vi "configure_tx_transfer_group.vi"(7 "Number of Groups":u16, 9 "Channels/Group":u16, 10 "Remote RDMA IP Address":string, 11 "Local RDMA IP Address":string) -> (3 "DSF Configuration":T1)   [LabVIEW 2020]
uses:
  <vilib>/addons/VeriStand Custom Device Scripting APIs/Data Sharing Framework/DSF Core.lvlibp/Typedefs/DSF Settings Info.ctl
  <vilib>/addons/VeriStand Custom Device Scripting APIs/Data Sharing Framework/DSF Core.lvlibp
  <vilib>/addons/VeriStand Custom Device Scripting APIs/Data Sharing Framework/DSF Core.lvlibp/Typedefs/DSF Data Type.ctl
  <vilib>/addons/VeriStand Custom Device Scripting APIs/Data Sharing Framework/DSF Core.lvlibp/Typedefs/Core Channel Configuration.ctl
  <vilib>/addons/VeriStand Custom Device Scripting APIs/Data Sharing Framework/DSF Core.lvlibp/Classes/Configuration/Core/Channel/Channel Configuration.lvclass
  <vilib>/addons/VeriStand Custom Device Scripting APIs/Data Sharing Framework/DSF Core.lvlibp/Typedefs/DSF Engine Channel Configuration.ctl
  <vilib>/addons/VeriStand Custom Device Scripting APIs/Data Sharing Framework/DSF Core.lvlibp/Typedefs/Core Transfer Configuration.ctl
  <vilib>/addons/VeriStand Custom Device Scripting APIs/Data Sharing Framework/DSF Core.lvlibp/Classes/Configuration/Core/Transfer/Transfer Configuration.lvclass
  <vilib>/addons/VeriStand Custom Device Scripting APIs/Data Sharing Framework/DSF Core.lvlibp/Typedefs/DSF Engine Transfer Configuration.ctl
  <vilib>/addons/VeriStand Custom Device Scripting APIs/Data Sharing Framework/DSF Core.lvlibp/Typedefs/DSF Timeout Behavior.ctl
  <vilib>/addons/VeriStand Custom Device Scripting APIs/Data Sharing Framework/DSF Core.lvlibp/Typedefs/DSF Timing Info.ctl
  <vilib>/addons/VeriStand Custom Device Scripting APIs/Data Sharing Framework/DSF Core.lvlibp/Typedefs/DSF Direction.ctl
  <vilib>/addons/VeriStand Custom Device Scripting APIs/Data Sharing Framework/DSF Core.lvlibp/Typedefs/Core Group Configuration.ctl
  <vilib>/addons/VeriStand Custom Device Scripting APIs/Data Sharing Framework/DSF Core.lvlibp/Classes/Configuration/Core/Group/Group Configuration.lvclass
  <vilib>/addons/VeriStand Custom Device Scripting APIs/Data Sharing Framework/DSF Core.lvlibp/Typedefs/DSF Engine Transfer Group Configuration.ctl
  <vilib>/addons/VeriStand Custom Device Scripting APIs/Data Sharing Framework/DSF Core.lvlibp/Typedefs/Core Thread Configuration.ctl
  <vilib>/addons/VeriStand Custom Device Scripting APIs/Data Sharing Framework/DSF Core.lvlibp/Classes/Configuration/Core/Thread/Thread Configuration.lvclass
  <vilib>/addons/VeriStand Custom Device Scripting APIs/Data Sharing Framework/DSF Core.lvlibp/Typedefs/DSF Engine Plugin Thread Configuration.ctl
  <vilib>/addons/VeriStand Custom Device Scripting APIs/Data Sharing Framework/DSF Core.lvlibp/Typedefs/Core Plugin Configuration.ctl
  <vilib>/addons/VeriStand Custom Device Scripting APIs/Data Sharing Framework/DSF Core.lvlibp/Classes/Configuration/Core/Plugin/Plugin Configuration.lvclass
  <vilib>/addons/VeriStand Custom Device Scripting APIs/Data Sharing Framework/DSF Core.lvlibp/Typedefs/DSF Engine Plugin Configuration.ctl
  <vilib>/addons/VeriStand Custom Device Scripting APIs/Data Sharing Framework/DSF Core.lvlibp/Typedefs/DSF Engine Framework Configuration.ctl
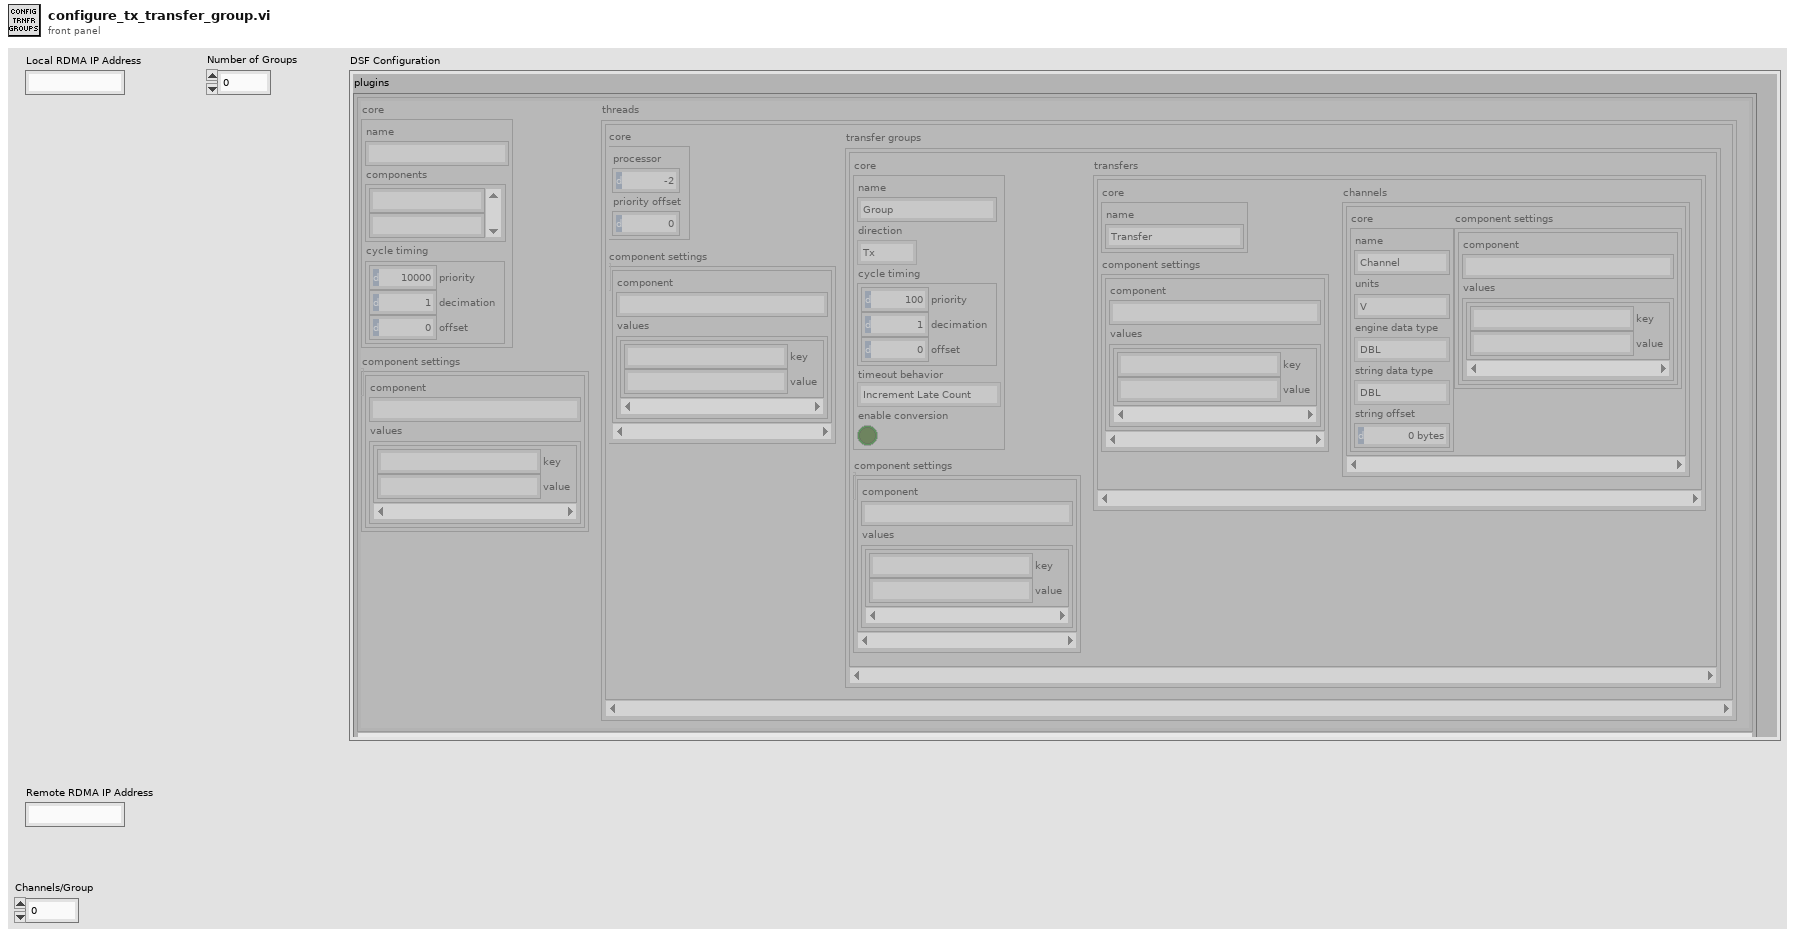
[diagram p1: front panel]
types:
  T1 = typedef "DSF Core.lvlibp/DSF Engine Framework Configuration.ctl" = cluster{"plugins":T2[]}
  T2 = typedef "DSF Core.lvlibp/DSF Engine Plugin Configuration.ctl" = cluster{"core":T3, "component settings":T5[], "threads":T6[]}
  T3 = typedef "DSF Core.lvlibp/Plugin Configuration.lvclass/Core Plugin Configuration.ctl" = cluster{"name":string, "components":string[], "cycle timing":T4}
  T4 = typedef "DSF Core.lvlibp/DSF Timing Info.ctl" = cluster{"priority":u64, "decimation":u64, "offset":u64}
  T5 = typedef "DSF Core.lvlibp/DSF Settings Info.ctl" = cluster{"component":string, "values":cluster{"key":string, "value":string}[]}
  T6 = typedef "DSF Core.lvlibp/DSF Engine Plugin Thread Configuration.ctl" = cluster{"core":T7, "component settings":T5[], "transfer groups":T8[]}
  T7 = typedef "DSF Core.lvlibp/Thread Configuration.lvclass/Core Thread Configuration.ctl" = cluster{"processor":i32, "priority offset":i16}
  T8 = typedef "DSF Core.lvlibp/DSF Engine Transfer Group Configuration.ctl" = cluster{"core":T9, "component settings":T5[], "transfers":T12[]}
  T9 = typedef "DSF Core.lvlibp/Group Configuration.lvclass/Core Group Configuration.ctl" = cluster{"name":string, "direction":T10, "cycle timing":T4, "timeout behavior":T11, "enable conversion":bool}
  T10 = typedef "DSF Core.lvlibp/DSF Direction.ctl" = enum8{"Tx", "Rx"}
  T11 = typedef "DSF Core.lvlibp/DSF Timeout Behavior.ctl" = enum8{"Increment Late Count", "Throw Error"}
  T12 = typedef "DSF Core.lvlibp/DSF Engine Transfer Configuration.ctl" = cluster{"core":T13, "component settings":T5[], "channels":T14[]}
  T13 = typedef "DSF Core.lvlibp/Transfer Configuration.lvclass/Core Transfer Configuration.ctl" = cluster{"name":string}
  T14 = typedef "DSF Core.lvlibp/DSF Engine Channel Configuration.ctl" = cluster{"core":T15, "component settings":T5[]}
  T15 = typedef "DSF Core.lvlibp/Channel Configuration.lvclass/Core Channel Configuration.ctl" = cluster{"name":string, "units":string, "engine data type":T16, "string data type":T16, "string offset":u64}
  T16 = typedef "DSF Core.lvlibp/DSF Data Type.ctl" = enum8{"Bool", "SGL", "DBL", "I8", "I16", "I32", "I64", "U8", "U16", "U32", "U64"}
  T17 = cluster{"component":string, "values":cluster{"key":string, "value":string}[]}[]
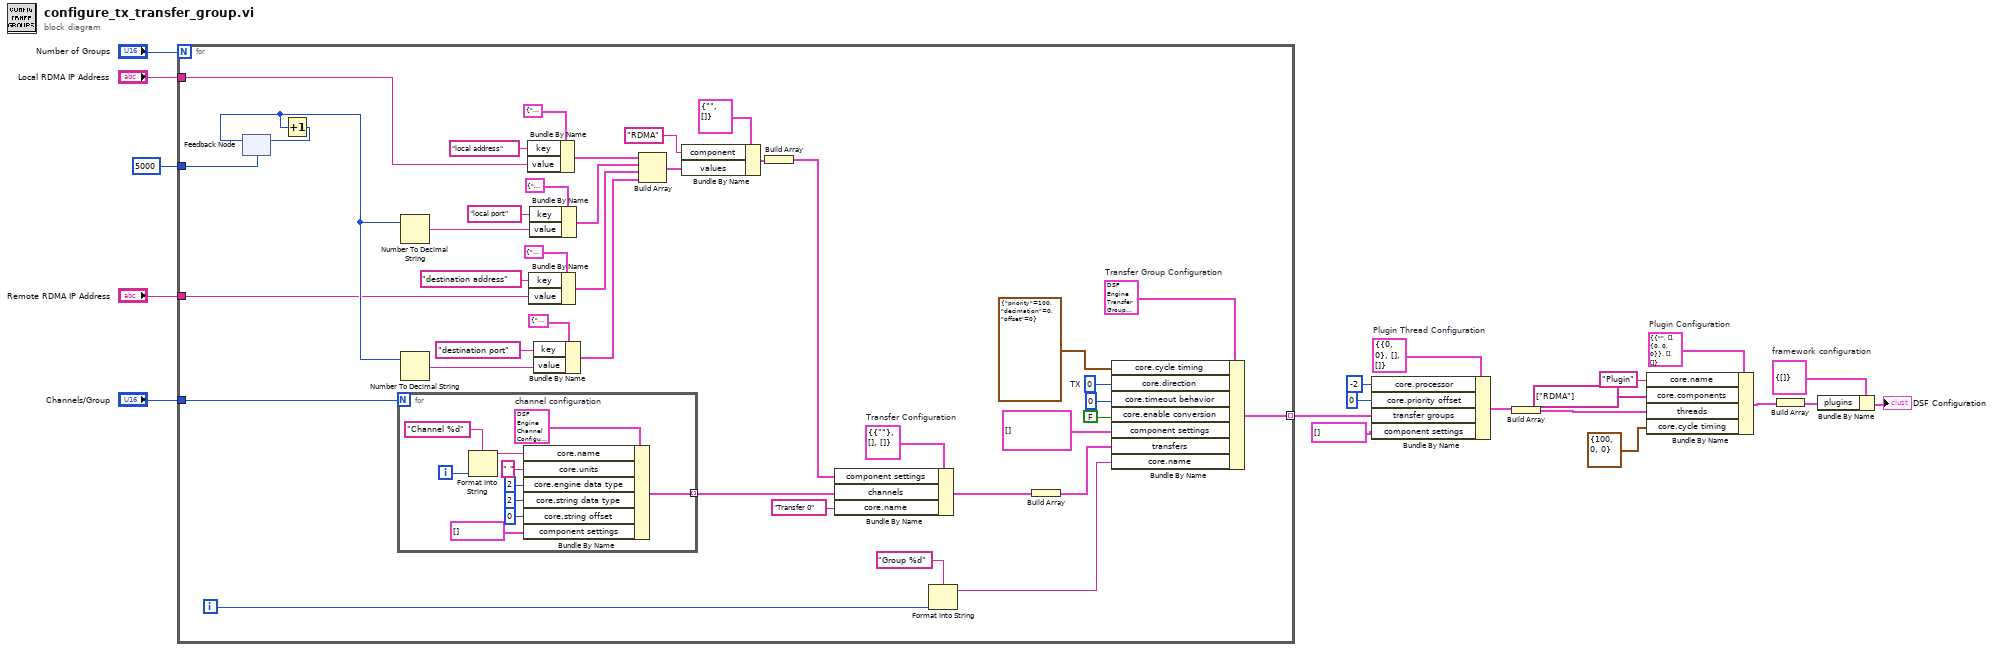
[diagram p0: block diagram]
diagram:
  w4 = T1 {"plugins"=[]}  # framework configuration
  w6 = T2 {"core"={"name"="", "components"=[], "cycle timing"={"priority"=0, "decimation"=0, "offset"=0}}, "component settings"=[], "threads"=[]}  # Plugin Configuration
  w12 = T6 {"core"={"processor"=0, "priority offset"=0}, "component settings"=[], "transfer groups"=[]}  # Plugin Thread Configuration
  n1 = for {
    N: "Number of Groups" -> [_]
    tunnel: [w54] -> w11 mode=indexing
    tunnel: u16 5000 ("Base port (5000)") -> [w52]
    tunnel: "Channels/Group" -> [w51]
    tunnel: "Local RDMA IP Address" -> [w22]
    tunnel: "Remote RDMA IP Address" -> [w21]
    i -> [w25]
    w32 = T12 {"core"={"name"=""}, "component settings"=[], "channels"=[]}  # Transfer Configuration
    w60 = T8 {"core"={"name"="", "direction"=enum."Tx", "cycle timing"={"priority"=0, "decimation"=0, "offset"=0}, "timeout behavior"=enum."Increment Late Count", "enable conversion"=FALSE}, "component settings"=[], "transfers"=[]}  # Transfer Group Configuration
    w56 = u32 0  # TX
    n2 = feedback #1(w52) -> (w30:u16)
    n3 = Increment(x=w30) -> (x+1=w29:u16)
    n4 = feedback-in #1(w29) -> ()
    n5 = for {
      N: w51 -> [_]
      tunnel: [w70] -> w28 mode=indexing
      i -> [w68]
      w61 = T14 {"core"={"name"="Channel", "units"="V", "engine data type"=enum."DBL", "string data type"=enum."DBL", "string offset"=0}, "component settings"=[]}  # channel configuration
      n6 = Format Into String(format string="Channel %d", w68) -> (resulting string=w67:string)  [unwired: 2 in, 1 out]
      n7 = Bundle By Name(cluster=w61, "core.name"=w67, "core.units"=" ", "core.engine data type"=u8 2, "core.string data type"=u8 2, "core.string offset"=u8 0, "component settings"=T17 []) -> (w70:T14)
    }
    n8 = Number To Decimal String(number=w30) -> (decimal integer string=w45:string)  [unwired: 1 in]
    n9 = Number To Decimal String(number=w30) -> (decimal integer string=w44:string)  [unwired: 1 in]
    n10 = Bundle By Name(cluster=cluster{"key":string, "value":string} {"key"="", "value"=""} ("value"), "key"="local address", "value"=w22) -> (w39:cluster{"key":string, "value":string})
    n11 = Bundle By Name(cluster=cluster{"key":string, "value":string} {"key"="", "value"=""} ("value"), "key"="destination address", "value"=w21) -> (w37:cluster{"key":string, "value":string})
    n12 = Bundle By Name(cluster=cluster{"key":string, "value":string} {"key"="", "value"=""} ("value"), "key"="local port", "value"=w45) -> (w38:cluster{"key":string, "value":string})
    n13 = Bundle By Name(cluster=cluster{"key":string, "value":string} {"key"="", "value"=""} ("value"), "key"="destination port", "value"=w44) -> (w36:cluster{"key":string, "value":string})
    n14 = Build Array(w39, w38, w37, w36) -> (w35:cluster{"key":string, "value":string}[])
    n15 = Bundle By Name(cluster=T5 {"component"="", "values"=[]} ("component settings"), "component"="RDMA", "values"=w35) -> (w34:T5)
    n16 = Build Array(w34) -> (w33:T5[])
    n17 = Bundle By Name(cluster=w32, "component settings"=w33, "channels"=w28, "core.name"="Transfer 0") -> (w55:T12)
    n18 = Format Into String(format string="Group %d", w25) -> (resulting string=w23:string)  [unwired: 2 in, 1 out]
    n19 = Build Array(w55) -> (w24:T12[])
    n20 = Bundle By Name(cluster=w60, "core.cycle timing"=T4 {"priority"=100, "decimation"=0, "offset"=0}, "core.direction"=w56, "core.timeout behavior"=u32 0, "core.enable conversion"=FALSE, "component settings"=T5[] [], "transfers"=w24, "core.name"=w23) -> (w54:T8)
  }
  n21 = Bundle By Name(cluster=w12, "core.processor"=-2, "core.priority offset"=0, "transfer groups"=w11, "component settings"=T17 []) -> (w10:T6)
  n22 = Build Array(w10) -> (w7:T6[])
  n23 = Bundle By Name(cluster=w6, "core.name"="Plugin", "core.components"=string[] ["RDMA"], "threads"=w7, "core.cycle timing"=T4 {"priority"=100, "decimation"=0, "offset"=0}) -> (w3:T2)
  n24 = Build Array(w3) -> (w5:T2[])
  n25 = Bundle By Name(cluster=w4, "plugins"=w5) -> (→"DSF Configuration":T1)
